vi "waveform gen.vi"(1 "Boolean":bool, 2 "galvo phase":dbl=89.0, 3 "Exposure Time (s)":dbl(ring)=0.5 items=["0.2"=0.2, "0.5"=0.5, "1.0"=1.0, "4.0"=4.0, "8.0"=8.0], 4 "Laser Power%(0-100)":dbl=10.0) -> (0 "waveform":waveform(dbl)[](array[waveform]))   [LabVIEW 2018]
uses:
  <vilib>/Analysis/coordinate.llb/2D Cartesian Coordinate Rotation (Array).vi
  <vilib>/measure/NI_MABase.lvlib
  <vilib>/Analysis/NI_AALPro.lvlib
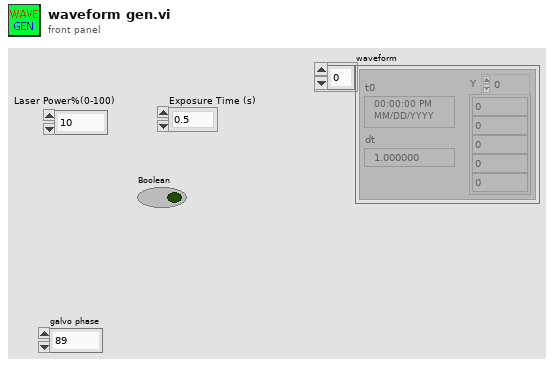
[diagram p1: front panel]
types:
  T1 = cluster{"Galvo/Pockels Cell Sampling Info":dbl, "#s":dbl}
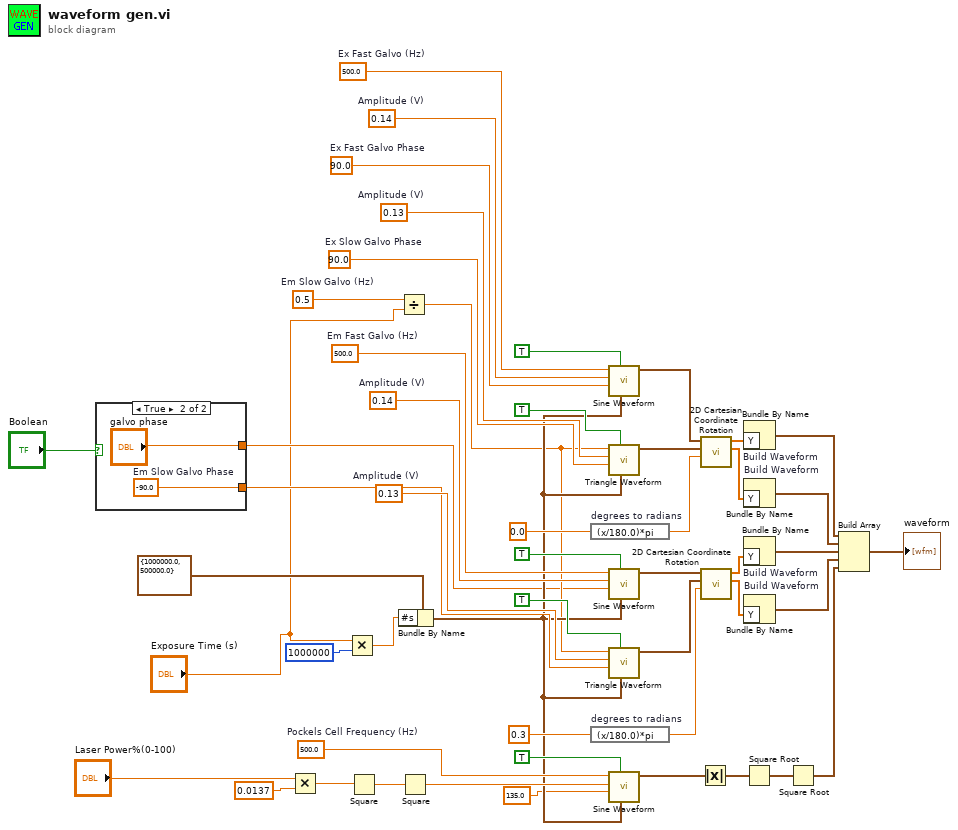
[diagram p0: block diagram]
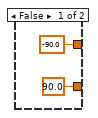
[diagram p2: hidden frame]
diagram:
  w8 = 0.5  # Em Slow Galvo (Hz)
  w39 = 0.13  # Amplitude (V)
  w49 = 0.13  # Amplitude (V)
  w48 = 500.0  # Ex Fast Galvo (Hz)
  w47 = 0.14  # Amplitude (V)
  w46 = 500.0  # Pockels Cell Frequency (Hz)
  w50 = 0.14  # Amplitude (V)
  w44 = 500.0  # Em Fast Galvo (Hz)
  w40 = 90.0  # Ex Slow Galvo Phase
  w41 = 90.0  # Ex Fast Galvo Phase
  n1 = case shown="True" "Boolean" {
    tunnel: [90.0 ("Em Slow Galvo Phase") w55] -> w13
    tunnel: [-90.0 ("Em Fast Galvo Phase") "galvo phase"] -> w5
    frame False {
    }
    frame True {
      w55 = -90.0  # Em Slow Galvo Phase
    }
  }
  n2 = Multiply(x="Laser Power%(0-100)", y=0.0137 ("data")) -> (x*y=w45:dbl)
  n3 = Multiply(x="Exposure Time (s)", y=1000000) -> (x*y=w9:dbl)
  n4 = Square(x=w45) -> (x^2=w32:dbl)
  n5 = Divide(x=w8, y="Exposure Time (s)") -> (x/y=w7:dbl)
  n6 = Bundle By Name(cluster=T1 {"Galvo/Pockels Cell Sampling Info"=1000000.0, "#s"=500000.0} ("Sampling Info"), "#s"=w9) -> (w11:T1)
  n7 = Square(x=w32) -> (x^2=w31:dbl)
  n8 = expression code="(x/180.0)*pi" "degrees to radians"(0.0 ("Ex Theta")) -> (w17:dbl)
  n9 = expression code="(x/180.0)*pi" "degrees to radians"(0.3 ("Em Theta")) -> (w14:dbl)
  n10 = call <vilib>:"Sine Waveform.vi"("sampling info"=w11, "reset signal"=TRUE, "phase"=w41, "amplitude"=w47, "frequency"=w48) -> ("signal out"=w29:waveform(dbl))  [unwired: 5 in, 1 out]
  n11 = call <vilib>:"Triangle Waveform.vi"("sampling info"=w11, "reset signal"=TRUE, "phase"=w40, "amplitude"=w49, "frequency"=w7) -> ("signal out"=w30:waveform(dbl))  [unwired: 5 in, 1 out]
  n12 = call <vilib>:"Sine Waveform.vi"("sampling info"=w11, "reset signal"=TRUE, "phase"=w5, "amplitude"=w50, "frequency"=w44) -> ("signal out"=w16:waveform(dbl))  [unwired: 5 in, 1 out]
  n13 = call <vilib>:"Triangle Waveform.vi"("sampling info"=w11, "reset signal"=TRUE, "phase"=w13, "amplitude"=w39, "frequency"=w7) -> ("signal out"=w21:waveform(dbl))  [unwired: 5 in, 1 out]
  n14 = call <vilib>:"Sine Waveform.vi"("sampling info"=w11, "reset signal"=TRUE, "phase"=135.0, "amplitude"=w31, "frequency"=w46) -> ("signal out"=w43:waveform(dbl))  [unwired: 5 in, 1 out]
  n15 = Absolute Value(x=w43) -> (abs(x)=w34:waveform(dbl))
  n16 = call-poly <vilib>:"2D Cartesian Coordinate Rotation.vi"("theta"=w17, "Y"=w30, "X"=w29) -> ("Y Out"=w26:dbl[], "X Out"=w28:dbl[])  [unwired: 6 in, 1 out]
  n17 = call-poly <vilib>:"2D Cartesian Coordinate Rotation.vi"("theta"=w14, "Y"=w21, "X"=w16) -> ("Y Out"=w22:dbl[], "X Out"=w23:dbl[])  [unwired: 6 in, 1 out]
  n18 = Bundle By Name "Build Waveform"("Y"=w28) -> (w27:waveform(dbl))  [unwired: 1 in]
  n19 = Bundle By Name "Build Waveform"("Y"=w26) -> (w25:waveform(dbl))  [unwired: 1 in]
  n20 = Bundle By Name "Build Waveform"("Y"=w23) -> (w19:waveform(dbl))  [unwired: 1 in]
  n21 = Bundle By Name "Build Waveform"("Y"=w22) -> (w20:waveform(dbl))  [unwired: 1 in]
  n22 = Square Root(x=w34) -> (sqrt(x)=w33:waveform(dbl))
  n23 = Square Root(x=w33) -> (sqrt(x)=w24:waveform(dbl))
  n24 = Build Array "Build Array"(w27, w25, w19, w20, w24) -> (→"waveform":waveform(dbl)[])
